vi "Rohde & Schwarz VNA Read Sweep Type.vi"(6 "Channel":i8=1 min=1 max=99 step=1, 7 "Rohde & Schwarz VNA":T1, 8 "error in (no error)":errorcluster, 11 "VISA Resource Name":refnum<visa-resource-name>) -> (0 "error out":errorcluster, 2 "Sweep Type":T2, 3 "dup VISA Resource Name":refnum<visa-resource-name>)   [LabVIEW 2011]
doc: "This VI for the HP 8753 is used to read the sweep type.\n\n0 LINEAR FREQ\n1 LOG FREQ\n2 LIST FREQ\n3 CW TIME\n4 POWER SWEEP"
uses:
  TypeDefs/Rohde & Schwarz VNA Sweep Type.ctl
  TypeDefs/Rohde & Schwarz VNA Instrument Info.ctl
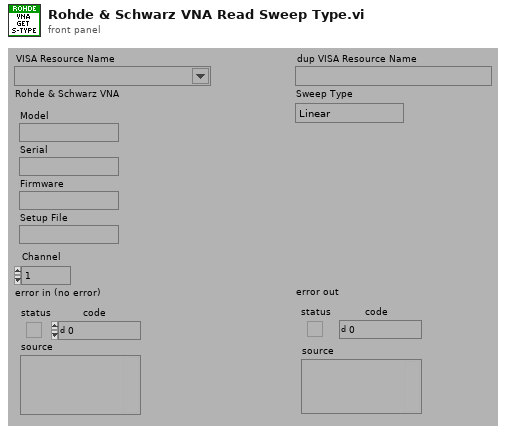
[diagram p1: front panel]
types:
  T1 = typedef "Rohde & Schwarz VNA Instrument Info.ctl" = cluster{"Model":string, "Serial":string, "Firmware":string, "Setup File":string}
  T2 = typedef "Rohde & Schwarz VNA Sweep Type.ctl" = enum32{"Linear", "Logarithmic", "Segmented", "Power", "Time", "CW"}
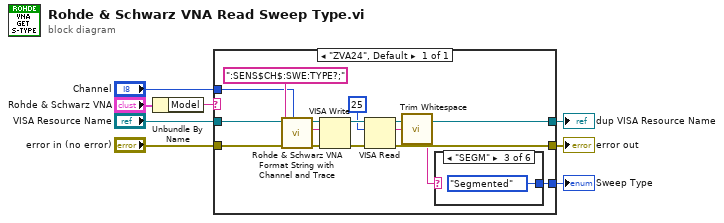
[diagram p0: block diagram]
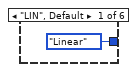
[diagram p2: hidden frame]
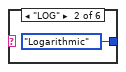
[diagram p3: hidden frame]
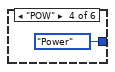
[diagram p4: hidden frame]
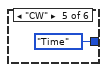
[diagram p5: hidden frame]
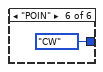
[diagram p6: hidden frame]
diagram:
  n1 = Unbundle By Name("Rohde & Schwarz VNA") -> ("Model"=w1:string)
  n2 = case shown="\"ZVA24\", Default" w1 {
    tunnel: "VISA Resource Name" -> [w17]
    tunnel: "error in (no error)" -> [w21]
    tunnel: [w20] -> w7
    tunnel: [w14] -> w6
    tunnel: [w15] -> w4
    tunnel: "Channel" -> [w9]
    frame "ZVA24", Default {
      n3 = call "Rohde & Schwarz VNA Format String with Channel and Trace.vi"("Channel"=w9, "String"=":SENS$CH$:SWE:TYPE?;") -> ("String Out"=w10:string)  [unwired: 1 in, 6 out]
      n4 = VISA Write(VISA resource name=w17, write buffer=w10, error in (no error)=w21) -> (VISA resource name out=w18:refnum<visa-resource-name>, error out=w19:errorcluster)  [unwired: 1 out]
      n5 = VISA Read(VISA resource name=w18, byte count=u32 25, error in (no error)=w19) -> (VISA resource name out=w15:refnum<visa-resource-name>, read buffer=w13:string, error out=w20:errorcluster)  [unwired: 1 out]
      n6 = call <vilib>:"Trim Whitespace.vi"("string"=w13) -> ("trimmed string"=w12:string)  [unwired: 1 in]
      n7 = case shown="\"SEGM\"" w12 {
        tunnel: [Rohde_&_Schwarz_VNA_Sweep_Type."Linear" ("sweep type") Rohde_&_Schwarz_VNA_Sweep_Type."Logarithmic" ("sweep type") Rohde_&_Schwarz_VNA_Sweep_Type."Segmented" ("sweep type") Rohde_&_Schwarz_VNA_Sweep_Type."Power" ("sweep type") Rohde_&_Schwarz_VNA_Sweep_Type."Time" ("sweep type") Rohde_&_Schwarz_VNA_Sweep_Type."CW" ("sweep type")] -> w14
        frame "LIN", Default {
        }
        frame "LOG" {
        }
        frame "SEGM" {
        }
        frame "POW" {
        }
        frame "CW" {
        }
        frame "POIN" {
        }
      }
    }
  }
  "Sweep Type" <- w6
  "dup VISA Resource Name" <- w4
  "error out" <- w7
